vi "Start Acquisition.vi"(0 "fpga interface in":refnum<k20>, 11 "error in (no error)":errorcluster) -> (4 "fpga interface out":refnum<k20>, 15 "error out":errorcluster)   [LabVIEW 2023, in "GettingStarted_Acq_148X_Host.lvlib"]
uses:
  GettingStarted_Acq_148X_Host.lvlib
  <instrlib>/FlexRIO/CSI-2/v2/FPGA/Types/Global Acquisition Engine State.ctl
  Types/148x_Acq_FPGA_Reference.ctl
  <vilib>/Utility/error.llb/Error Cluster From Error Code.vi
  <vilib>/rvi/errors/niLvFpgaAdjustHostInterfaceError.vi
  <vilib>/rvi/interface/nirviReadWriteControl/nirviReadWriteControl.xnode
  <instrlib>/FlexRIO/CSI-2/v2/FPGA/NI CSI-2 API FPGA v2.lvlib
  NiFpgaLv.dll
  <vilib>/rvi/interface/Simulation/niFpgaSimulationCallBeginRW.vi
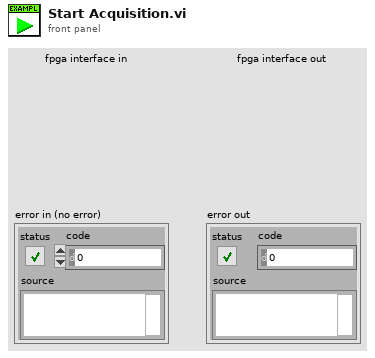
[diagram p1: front panel]
types:
  T1 = typedef "NI CSI-2 API FPGA v2.lvlib/Global Acquisition Engine State.ctl" = enum8{"Idle", "Ready For Start Trigger", "Acquire", "Error"}
  T2 = typedef "GettingStarted_Acq_148X_Host.lvlib/148x_Acq_FPGA_Reference.ctl" = refnum<k20>
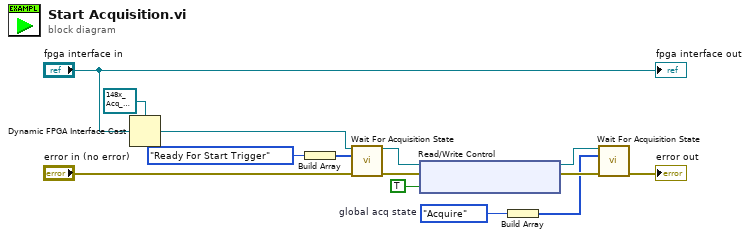
[diagram p0: block diagram]
diagram:
  w14 = Global_Acquisition_Engine_State."Acquire"  # global acq state
  n1 = Dynamic FPGA Interface Cast(Session In=T2 refnum ("FPGA VI Reference Out"), Type="fpga interface in") -> (Session Out=w4:T2)
  n2 = Build Array(Global_Acquisition_Engine_State."Ready For Start Trigger" ("global acq state")) -> (w2:T1[])
  n3 = call "Wait For Acquisition State.vi"("fpga interface in"=w4, "global acq state"=w2, "error in (no error)"="error in (no error)") -> ("fpga interface out"=w5:T2, "error out"=w6:errorcluster)  [unwired: 11 in]
  n4 = xnode "Read/Write Control"("FPGA VI Reference In"=w5, "error in"=w6, "sw start trigger (strobe)"=TRUE ("start trigger (strobe)")) -> ("FPGA VI Reference Out"=w10:T2, "error out"=w11:errorcluster)
  n5 = Build Array(w14) -> (w1:T1[])
  n6 = call "Wait For Acquisition State.vi"("fpga interface in"=w10, "global acq state"=w1, "error in (no error)"=w11) -> ("error out"=→"error out":errorcluster)  [unwired: 11 in, 1 out]
  "fpga interface out" <- "fpga interface in"
